vi "DriveGlobals.vi"() -> ()   [LabVIEW 2020]
panel:
  in  "EncoderDistance(Left)":dbl
  in  "EncoderDistance(Right)":dbl
  in  "EncoderSpeed(Left)":dbl
  in  "EncoderSpeed(Right)":dbl
  in  "LimitLeftSpeedDemand":dbl
  in  "LimitRightSpeedDemand":dbl
  in  "LeftSpeedDemand":dbl
  in  "RightSpeedDemand":dbl
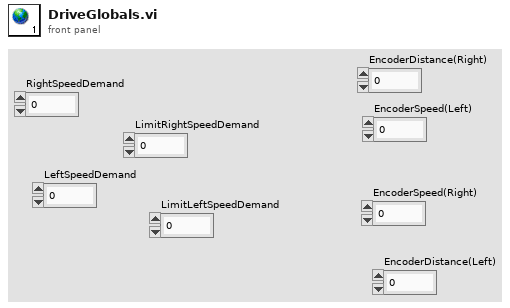
[diagram p1: front panel]
diagram:
